vi "ReadTerminal.vi"(1 "reference":refnum<vi>) -> (0 "Terminal":T4)   [LabVIEW 2013]
uses:
  <vilib>/Utility/miscctls.llb/LVBoundsTypeDef.ctl
  <vilib>/Utility/miscctls.llb/LVPositionTypeDef.ctl
  <vilib>/Utility/miscctls.llb/LVRectTypeDef.ctl
panel:
  out "error out 21":errorcluster
  out "error out 20":errorcluster
  out "error out 19":errorcluster
  out "error out 18":errorcluster
  out "error out 17":errorcluster
  out "error out 16":errorcluster
  out "error out 15":errorcluster
  out "error out 14":errorcluster
  out "error out 13":errorcluster
  out "error out 12":errorcluster
  out "error out 11":errorcluster
  out "error out 10":errorcluster
  out "error out 9":errorcluster
  out "error out 8":errorcluster
  out "error out 7":errorcluster
  out "error out 6":errorcluster
  out "error out 5":errorcluster
  out "error out 4":errorcluster
  out "error out 3":errorcluster
  out "error out 2":errorcluster
  out "error out":errorcluster
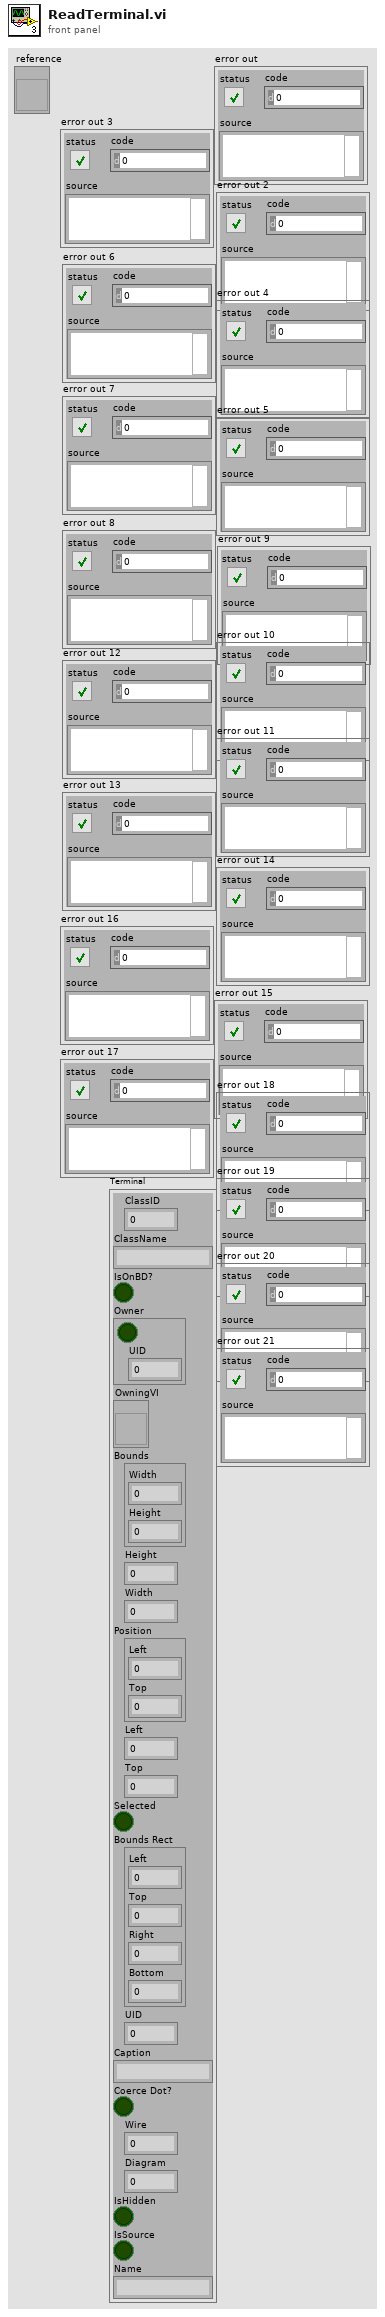
[diagram p1: front panel]
types:
  T1 = typedef "LVBoundsTypeDef.ctl" = cluster{"Width":u32, "Height":u32}
  T2 = typedef "LVPositionTypeDef.ctl" = cluster{"Left":i32, "Top":i32}
  T3 = typedef "LVRectTypeDef.ctl" = cluster{"Left":i16, "Top":i16, "Right":i16, "Bottom":i16}
  T4 = cluster{"ClassID":u32, "ClassName":string, "IsOnBD?":bool, "Owner":cluster{bool, "UID":i32}, "OwningVI":refnum<vi>, "Bounds":T1, "Height":u32, "Width":u32, "Position":T2, "Left":i32, "Top":i32, "Selected":bool, "Bounds Rect":T3, "UID":i32, "Caption":string, "Coerce Dot?":bool, "Wire":i32, "Diagram":i32, "IsHidden":bool, "IsSource":bool, "Name":string}
  T5 = cluster{"ClassID":u32, "ClassName":string, "IsOnBD?":bool, "Cluster":cluster{bool, "UID":i32}, "OwningVI":refnum<vi>, "Bounds":T1, "Height":u32, "Width":u32, "Position":T2, "Left":i32, "Top":i32, "Selected":bool, "Bounds Rect":T3, "UID":i32, "Caption":string, "Coerce Dot?":bool, "UID":i32, "UID":i32, "IsHidden":bool, "IsSource":bool, "Name":string}
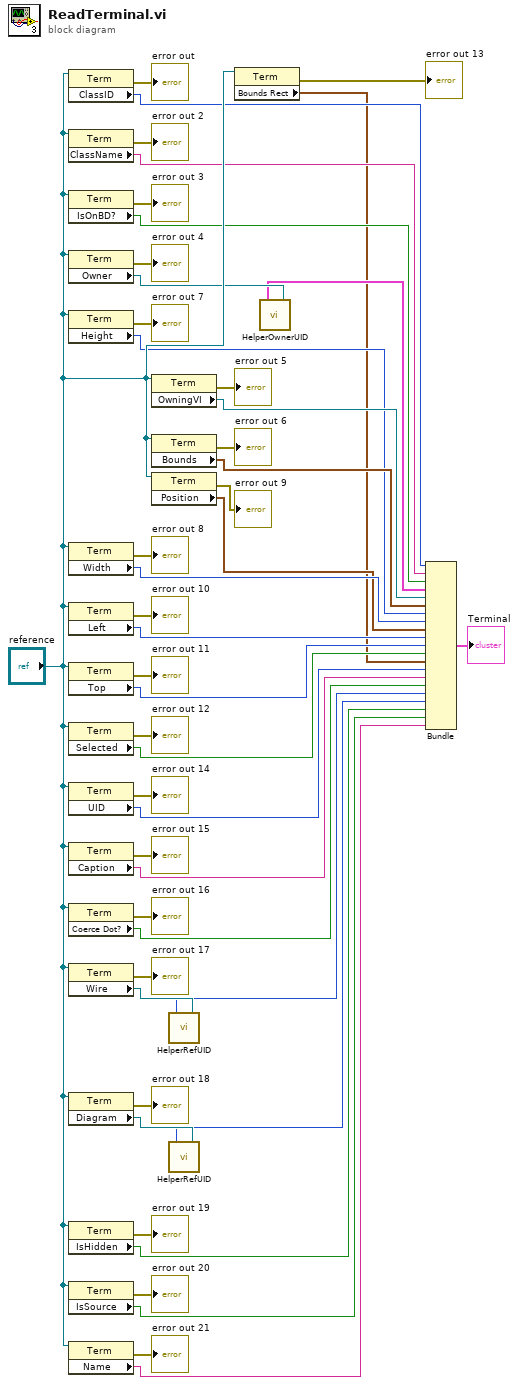
[diagram p0: block diagram]
diagram:
  n1 = property class="Term"(reference="reference") -> (error out=→"error out":errorcluster, "ClassID"=w45:u32)  [unwired: 1 in, 1 out]
  n2 = property class="Term"(reference="reference") -> (error out=→"error out 2":errorcluster, "ClassName"=w43:string)  [unwired: 1 in, 1 out]
  n3 = property class="Term"(reference="reference") -> (error out=→"error out 3":errorcluster, "IsOnBD?"=w41:bool)  [unwired: 1 in, 1 out]
  n4 = property class="Term"(reference="reference") -> (error out=→"error out 4":errorcluster, "Owner"=w39:refnum<vi>)  [unwired: 1 in, 1 out]
  n5 = property class="Term"(reference="reference") -> (error out=→"error out 7":errorcluster, "Height"=w32:u32)  [unwired: 1 in, 1 out]
  n6 = property class="Term"(reference="reference") -> (error out=→"error out 8":errorcluster, "Width"=w30:u32)  [unwired: 1 in, 1 out]
  n7 = property class="Term"(reference="reference") -> (error out=→"error out 10":errorcluster, "Left"=w26:i32)  [unwired: 1 in, 1 out]
  n8 = property class="Term"(reference="reference") -> (error out=→"error out 11":errorcluster, "Top"=w24:i32)  [unwired: 1 in, 1 out]
  n9 = property class="Term"(reference="reference") -> (error out=→"error out 12":errorcluster, "Selected"=w22:bool)  [unwired: 1 in, 1 out]
  n10 = property class="Term"(reference="reference") -> (error out=→"error out 14":errorcluster, "UID"=w18:i32)  [unwired: 1 in, 1 out]
  n11 = property class="Term"(reference="reference") -> (error out=→"error out 15":errorcluster, "Caption"=w16:string)  [unwired: 1 in, 1 out]
  n12 = property class="Term"(reference="reference") -> (error out=→"error out 16":errorcluster, "Coerce Dot?"=w14:bool)  [unwired: 1 in, 1 out]
  n13 = property class="Term"(reference="reference") -> (error out=→"error out 17":errorcluster, "Wire"=w12:refnum<vi>)  [unwired: 1 in, 1 out]
  n14 = property class="Term"(reference="reference") -> (error out=→"error out 18":errorcluster, "Diagram"=w9:refnum<vi>)  [unwired: 1 in, 1 out]
  n15 = property class="Term"(reference="reference") -> (error out=→"error out 19":errorcluster, "IsHidden"=w6:bool)  [unwired: 1 in, 1 out]
  n16 = property class="Term"(reference="reference") -> (error out=→"error out 20":errorcluster, "IsSource"=w4:bool)  [unwired: 1 in, 1 out]
  n17 = property class="Term"(reference="reference") -> (error out=→"error out 21":errorcluster, "Name"=w2:string)  [unwired: 1 in, 1 out]
  n18 = property class="Term"(reference="reference") -> (error out=→"error out 5":errorcluster, "OwningVI"=w36:refnum<vi>)  [unwired: 1 in, 1 out]
  n19 = property class="Term"(reference="reference") -> (error out=→"error out 6":errorcluster, "Bounds"=w34:T1)  [unwired: 1 in, 1 out]
  n20 = property class="Term"(reference="reference") -> (error out=→"error out 9":errorcluster, "Position"=w28:T2)  [unwired: 1 in, 1 out]
  n21 = call "HelperRefUID.vi"("Text in"=w12) -> ("UID"=w11:i32)
  n22 = call "HelperRefUID.vi"("Text in"=w9) -> ("UID"=w8:i32)
  n23 = property class="Term"(reference="reference") -> (error out=→"error out 13":errorcluster, "Bounds Rect"=w20:T3)  [unwired: 1 in, 1 out]
  n24 = call "HelperOwnerUID.vi"("Generic in"=w39) -> ("Cluster"=w38:cluster{bool, "UID":i32})
  n25 = Bundle("ClassID"=w45, "ClassName"=w43, "IsOnBD?"=w41, "Cluster"=w38, "OwningVI"=w36, "Bounds"=w34, "Height"=w32, "Width"=w30, "Position"=w28, "Left"=w26, "Top"=w24, "Selected"=w22, "Bounds Rect"=w20, "UID"=w18, "Caption"=w16, "Coerce Dot?"=w14, "UID"=w11, "UID"=w8, "IsHidden"=w6, "IsSource"=w4, "Name"=w2) -> (→"Terminal":T5)  [unwired: 1 in]
